vi "SEARCH DATA.vi"(11 "REFERENCES":T1) -> (3 "DATA OUT":string[][](array[string]))   [LabVIEW 2019]
uses:
  Controls/References Cluster.ctl
  Controls/Custom Calendar/Custom Calendar.xctl
  <vilib>/addons/database/Auxilliary.llb/DB Tools Cursor Type.ctl
  Controls/Column Names/Inventory Column Names.ctl
  Controls/Column Names/User Column Names.ctl
  Controls/Column Names/Inventory Archive Column Names.ctl
  Controls/Column Names/User Archive Column Names.ctl
  Controls/Column Names/Checked In Archive Column Names.ctl
  Controls/Column Names/Sales Tracking Column Names.ctl
  <vilib>/addons/database/Connection.llb/DB Tools Open Connec (String).vi
  <vilib>/addons/database/Connection.llb/Conn Execute.vi
  <vilib>/addons/database/Recordset.llb/Rec Fetch Recordset Data (R).vi
  <vilib>/addons/database/Recordset.llb/Rec Destroy - Connection.vi
  <vilib>/addons/database/_DB Variant To Data/Database Variant To Data.xnode
  <vilib>/addons/database/NI_Database_API.lvlib
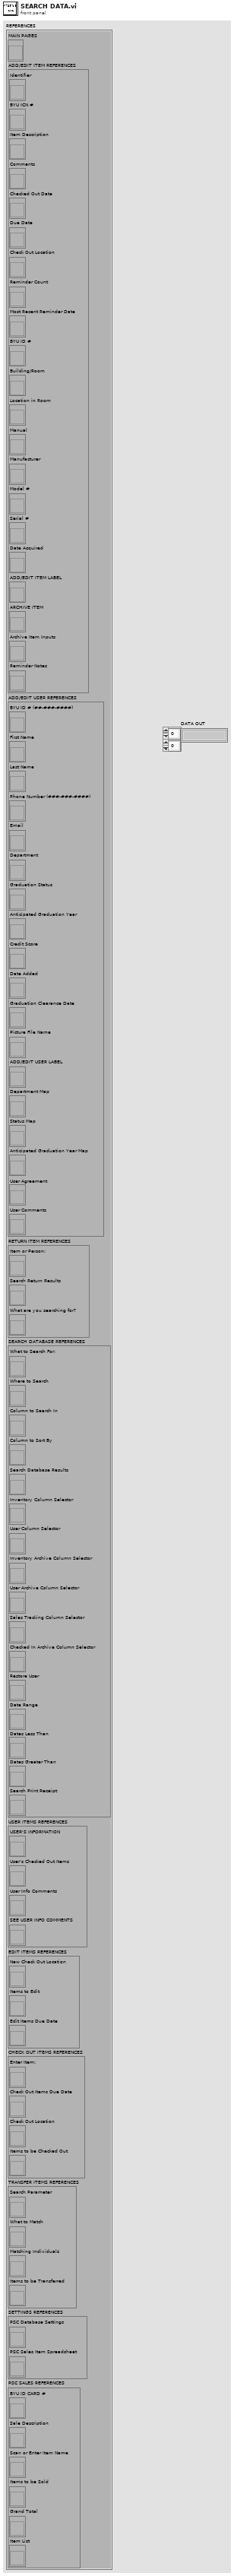
[diagram p1: front panel]
types:
  T1 = typedef "References Cluster.ctl" = cluster{"MAIN PAGES":refnum<vi>, "ADD/EDIT ITEM REFERENCES":cluster{"Identifier":refnum<vi>, "BYU ICN #":refnum<vi>, "Item Description":refnum<vi>, "Comments":refnum<vi>, "Checked Out Date":refnum<vi>, "Due Date":refnum<vi>, "Check Out Location":refnum<vi>, "Reminder Count":refnum<vi>, "Most Recent Reminder Date":refnum<vi>, "BYU ID #":refnum<vi>, "Building/Room":refnum<vi>, "Location in Room":refnum<vi>, "Manual":refnum<vi>, "Manufacturer":refnum<vi>, "Model #":refnum<vi>, "Serial #":refnum<vi>, "Date Acquired":refnum<vi>, "ADD/EDIT ITEM LABEL":refnum<vi>, "ARCHIVE ITEM":refnum<vi>, "Archive Item Inputs":refnum<vi>, "Reminder Notes":refnum<vi>}, "ADD/EDIT USER REFERENCES":cluster{"BYU ID # (##-###-####)":refnum<vi>, "First Name":refnum<vi>, "Last Name":refnum<vi>, "Phone Number (###-###-####)":refnum<vi>, "Email":refnum<vi>, "Department":refnum<vi>, "Graduation Status":refnum<vi>, "Anticipated Graduation Year":refnum<vi>, "Credit Score":refnum<vi>, "Date Added":refnum<vi>, "Graduation Clearance Date":refnum<vi>, "Picture File Name":refnum<vi>, "ADD/EDIT USER LABEL":refnum<vi>, "Department Map":refnum<vi>, "Status Map":refnum<vi>, "Anticipated Graduation Year Map":refnum<vi>, "User Agreement":refnum<vi>, "User Comments":refnum<vi>}, "RETURN ITEM REFERENCES":cluster{"Item or Person:":refnum<vi>, "Search Return Results":refnum<vi>, "What are you searching for?":refnum<vi>}, "SEARCH DATABASE REFERENCES":cluster{"What to Search For:":refnum<vi>, "Where to Search":refnum<vi>, "Column to Search In":refnum<vi>, "Column to Sort By":refnum<vi>, "Search Database Results":refnum<vi>, "Inventory Column Selector":refnum<vi>, "User Column Selector":refnum<vi>, "Inventory Archive Column Selector":refnum<vi>, "User Archive Column Selector":refnum<vi>, "Sales Tracking Column Selector":refnum<vi>, "Checked In Archive Column Selector":refnum<vi>, "Restore User":refnum<vi>, "Date Range":refnum<vi>, "Dates Less Than":refnum<vi>, "Dates Greater Than":refnum<vi>, "Search Print Receipt":refnum<vi>}, "USER ITEMS REFERENCES":cluster{"USER'S INFORMATION":refnum<vi>, "User's Checked Out Items":refnum<vi>, "User Info Comments":refnum<vi>, "SEE USER INFO COMMENTS":refnum<vi>}, "EDIT ITEMS REFERENCES":cluster{"New Check Out Location":refnum<vi>, "Items to Edit":refnum<vi>, "Edit Items Due Date":refnum<vi>}, "CHECK OUT ITEMS REFERENCES":cluster{"Enter Item:":refnum<vi>, "Check Out Items Due Date":refnum<vi>, "Check Out Location":refnum<vi>, "Items to be Checked Out":refnum<vi>}, "TRANSFER ITEMS REFERENCES":cluster{"Search Parameter":refnum<vi>, "What to Match":refnum<vi>, "Matching Individuals":refnum<vi>, "Items to be Transferred":refnum<vi>}, "SETTINGS REFERENCES":cluster{"PSC Database Settings":refnum<vi>, "PSC Sales Item Spreadsheet":refnum<vi>}, "PSC SALES REFERENCES":cluster{"BYU ID CARD #":refnum<vi>, "Sale Description":refnum<vi>, "Scan or Enter Item Name":refnum<vi>, "Items to be Sold":refnum<vi>, "Grand Total":refnum<vi>, "Item List":refnum<vi>}}
  T2 = cluster{"What to Search For:":refnum<vi>, "Where to Search":refnum<vi>, "Column to Search In":refnum<vi>, "Column to Sort By":refnum<vi>, "Search Database Results":refnum<vi>, "Inventory Column Selector":refnum<vi>, "User Column Selector":refnum<vi>, "Inventory Archive Column Selector":refnum<vi>, "User Archive Column Selector":refnum<vi>, "Sales Tracking Column Selector":refnum<vi>, "Checked In Archive Column Selector":refnum<vi>, "Restore User":refnum<vi>, "Date Range":refnum<vi>, "Dates Less Than":refnum<vi>, "Dates Greater Than":refnum<vi>, "Search Print Receipt":refnum<vi>}
  T3 = typedef "NI_Database_API.lvlib/Conn ObjectReference.ctl" = refnum<k1>
  T4 = typedef "Inventory Column Names.ctl" = string[]
  T5 = typedef "NI_Database_API.lvlib/DB Tools Cursor Type.ctl" = enum16{"forward-only", "keyset", "dynamic", "static"}
  T6 = enum8{"Enabled", "Disabled", "Disabled and Grayed Out"}
  T7 = typedef "User Column Names.ctl" = string[]
  T8 = typedef "Inventory Archive Column Names.ctl" = string[]
  T9 = typedef "User Archive Column Names.ctl" = string[]
  T10 = typedef "Checked In Archive Column Names.ctl" = string[]
  T11 = typedef "Sales Tracking Column Names.ctl" = string[]
  T12 = typedef "NI_Database_API.lvlib/Rec ObjectReference.ctl" = refnum<k1>
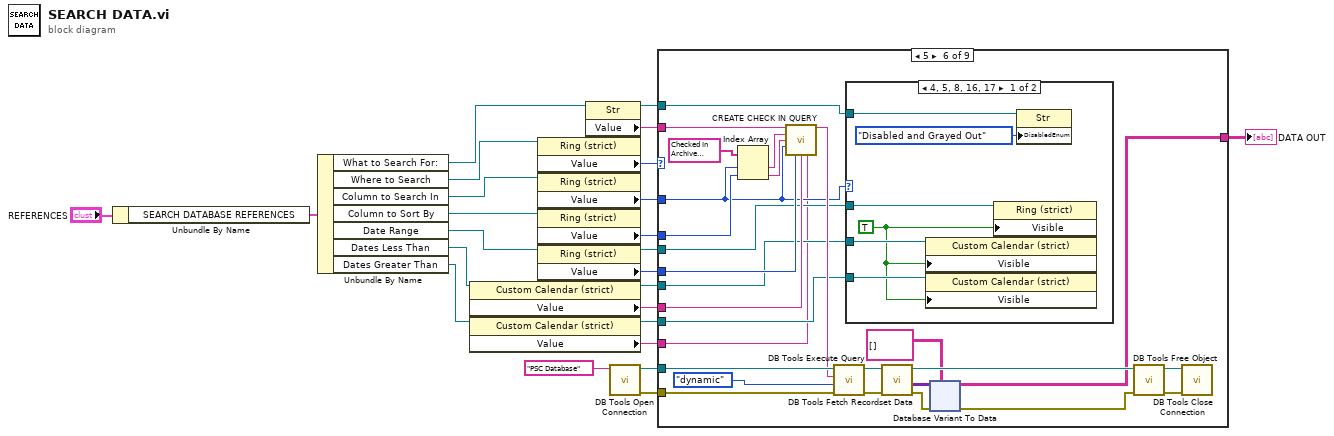
[diagram p0: block diagram]
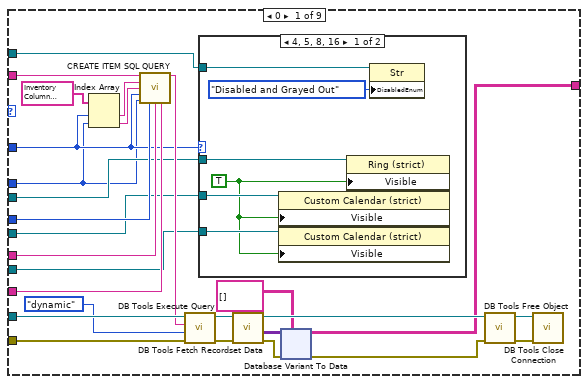
[diagram p2: hidden frame]
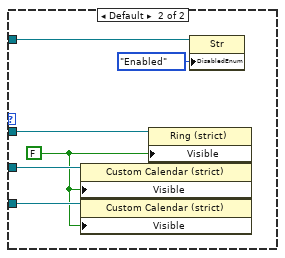
[diagram p3: hidden frame]
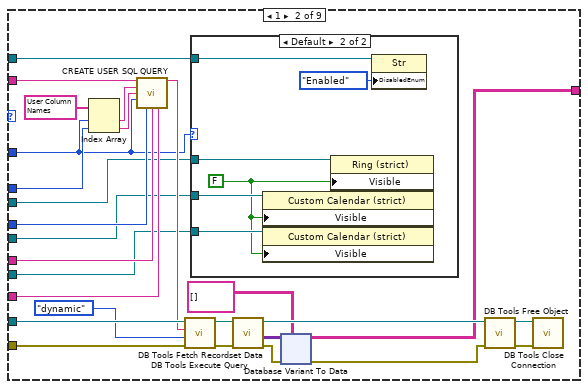
[diagram p4: hidden frame]
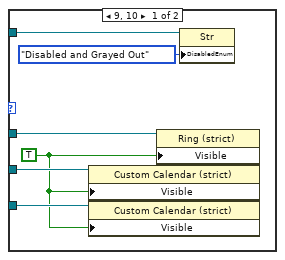
[diagram p5: hidden frame]
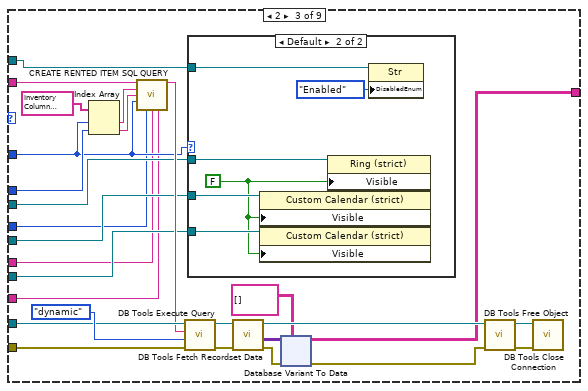
[diagram p6: hidden frame]
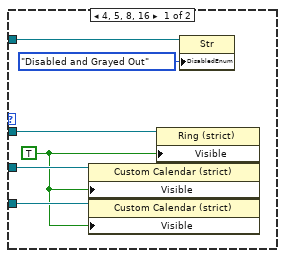
[diagram p7: hidden frame]
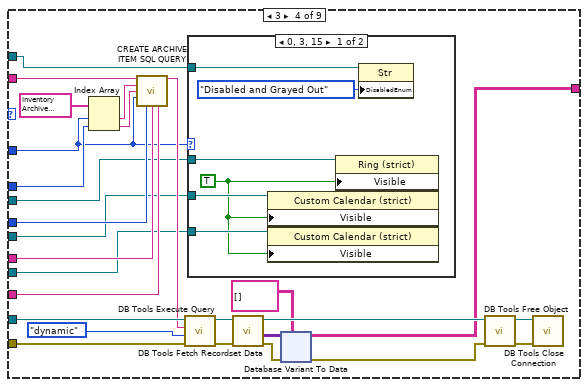
[diagram p8: hidden frame]
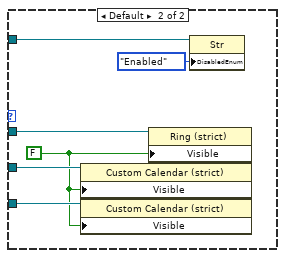
[diagram p9: hidden frame]
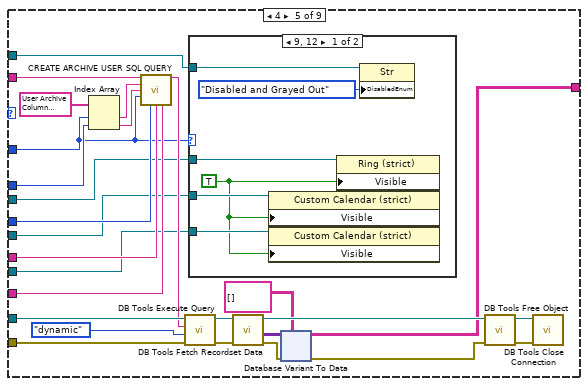
[diagram p10: hidden frame]
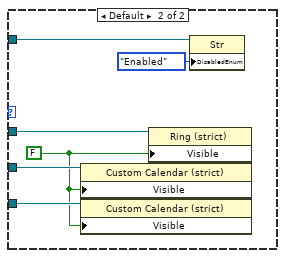
[diagram p11: hidden frame]
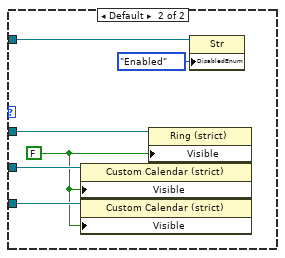
[diagram p12: hidden frame]
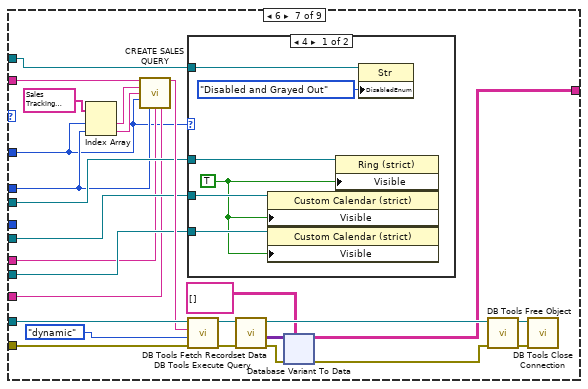
[diagram p13: hidden frame]
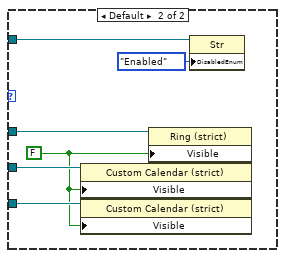
[diagram p14: hidden frame]
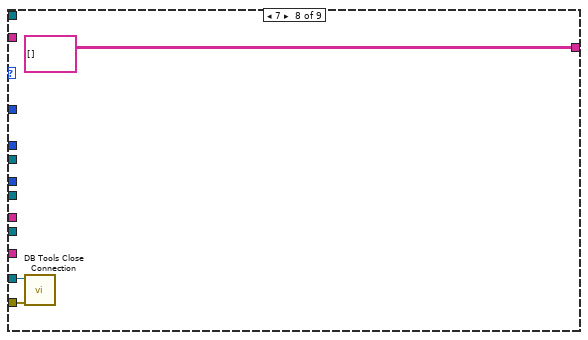
[diagram p15: hidden frame]
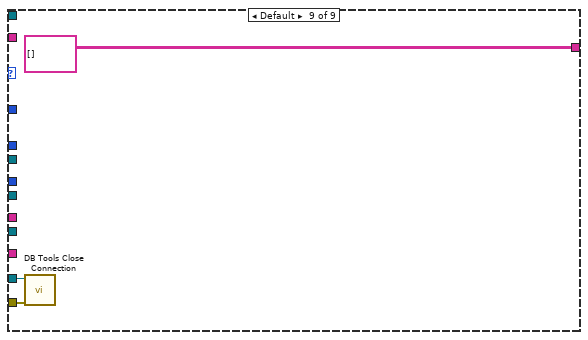
[diagram p16: hidden frame]
diagram:
  n1 = Unbundle By Name("REFERENCES") -> ("SEARCH DATABASE REFERENCES"=w13:T2)
  n2 = Unbundle By Name(w13) -> ("What to Search For:"=w18:refnum<vi>, "Where to Search"=w15:refnum<vi>, "Column to Search In"=w16:refnum<vi>, "Column to Sort By"=w17:refnum<vi>, "Date Range"=w10:refnum<vi>, "Dates Less Than"=w8:refnum<vi>, "Dates Greater Than"=w9:refnum<vi>)
  n3 = property class="Custom Calendar (strict)"(reference=w8) -> (reference out=w3:refnum<vi>, "Value"=w6:string)  [unwired: 1 in, 1 out]
  n4 = property class="Custom Calendar (strict)"(reference=w9) -> (reference out=w2:refnum<vi>, "Value"=w5:string)  [unwired: 1 in, 1 out]
  n5 = property class="Ring (strict)"(reference=w15) -> ("Value"=w24:u16)  [unwired: 1 in, 2 out]
  n6 = property class="Ring (strict)"(reference=w16) -> ("Value"=w23:u16)  [unwired: 1 in, 2 out]
  n7 = property class="Ring (strict)"(reference=w17) -> ("Value"=w22:u16)  [unwired: 1 in, 2 out]
  n8 = property class="Ring (strict)"(reference=w10) -> (reference out=w4:refnum<vi>, "Value"=w7:u16)  [unwired: 1 in, 1 out]
  n9 = property class="Str"(reference=w18) -> (reference out=w1:refnum<vi>, "Value"=w19:string)  [unwired: 1 in, 1 out]
  n10 = call-poly <vilib>:"DB Tools Open Connection.vi"("connection information"="PSC Database" ("string")) -> ("error out"=w20:errorcluster, "connection reference"=w21:T3)  [unwired: 7 in]
  n11 = case shown="5" w24 {
    tunnel: w23 -> [w31 w108 w195 w277 w361 w442 w523 _ _]
    tunnel: w22 -> [w25 w133 w217 w299 w383 w458 w526 _ _]
    tunnel: w21 -> [w51 w129 w210 w294 w376 w460 w538 w607 w610]
    tunnel: w20 -> [w50 w128 w209 w293 w375 w459 w537 w606 w609]
    tunnel: w19 -> [w43 w134 w216 w300 w382 w457 w548 _ _]
    tunnel: [w35 w118 w200 w284 w366 w450 w534 string[][] [] ("recordset data") string[][] [] ("recordset data")] -> w11
    tunnel: w7 -> [w34 w115 w194 w281 w364 w448 _ _ _]
    tunnel: w6 -> [w33 w114 w193 w280 w363 w447 w525 _ _]
    tunnel: w5 -> [w32 w113 w192 w279 w362 w441 w524 _ _]
    tunnel: w4 -> [w30 w111 w198 w276 w359 w445 w529 _ _]
    tunnel: w3 -> [w29 w110 w197 w275 w358 w444 w528 _ _]
    tunnel: w2 -> [w28 w109 w196 w274 w357 w443 w527 _ _]
    tunnel: w1 -> [w27 w112 w199 w278 w360 w446 w530 _ _]
    frame 0 {
      n12 = Index Array(array=T4 ["\"Identifier\"", "\"BYU ICN #\"", "\"Item Description\"", "\"Comments\"", "\"Checked Out Date\"", "\"Due Date\"", "\"Check Out Location\"", "\"Reminder Count\"", "\"Most Recent Reminder Date\"", "\"BYU ID #\"", "\"Building/Room\"", "\"Location in Room\"", "\"Manual\"", "\"Manufacturer\"", "\"Model #\"", "\"Serial #\"", "\"Date Acquired\"", "\"Reminder Notes\"", "\"First Name\"", "\"Last Name\""] ("INVENTORY COLUMN NAMES"), index #1=w31, index #2=w25) -> (element #1=w41:string, element #2=w40:string)
      n13 = call "CREATE ITEM SQL QUERY.vi"("What to Search"=w43, "Search Column Name"=w41, "Sorting Column Name"=w40, "Column to Search In"=w31, "Column to Sort By"=w25, "Date Range"=w34, "Dates Less Than"=w33, "Dates Greater Than"=w32) -> ("SQL QUERY"=w42:string)  [unwired: 7 in]
      n14 = call-poly <vilib>:"DB Tools Execute Query.vi"("error in (no error)"=w50, "cursor type"=DB_Tools_Cursor_Type."dynamic", "SQL query"=w42, "connection reference"=w51) -> ("error out"=w47:errorcluster, "recordset reference"=w48:T12)  [unwired: 4 in]
      n15 = case shown="4, 5, 8, 16" w31 {
        tunnel: w30 -> [w55 w61]
        tunnel: w29 -> [w56 w62]
        tunnel: w28 -> [w57 w63]
        tunnel: w27 -> [w53 w59]
        frame 4, 5, 8, 16 {
          w54 = TRUE ("Visible")
          n16 = property class="Custom Calendar (strict)"(reference=w56, "Visible"=w54) -> ()  [unwired: 1 in, 2 out]
          n17 = property class="Custom Calendar (strict)"(reference=w57, "Visible"=w54) -> ()  [unwired: 1 in, 2 out]
          n18 = property class="Ring (strict)"(reference=w55, "Visible"=w54) -> ()  [unwired: 1 in, 2 out]
          n19 = property class="Str"(reference=w53, "DisabledEnum"=T6."Disabled and Grayed Out" ("Disabled")) -> ()  [unwired: 1 in, 2 out]
        }
        frame Default {
          w58 = FALSE ("Visible")
          n20 = property class="Custom Calendar (strict)"(reference=w62, "Visible"=w58) -> ()  [unwired: 1 in, 2 out]
          n21 = property class="Custom Calendar (strict)"(reference=w63, "Visible"=w58) -> ()  [unwired: 1 in, 2 out]
          n22 = property class="Ring (strict)"(reference=w61, "Visible"=w58) -> ()  [unwired: 1 in, 2 out]
          n23 = property class="Str"(reference=w59, "DisabledEnum"=T6."Enabled" ("Disabled")) -> ()  [unwired: 1 in, 2 out]
        }
      }
      n24 = call-poly <vilib>:"DB Tools Fetch Recordset Data.vi"("error in (no error)"=w47, "recordset reference"=w48) -> ("error out"=w38:errorcluster, "recordset data"=w39:variant[][], "recordset reference out"=w46:T12)  [unwired: 3 in]
      n25 = xnode "Database Variant To Data"("database variant"=w39, "error in (no error)"=w38, "type"=string[][] []) -> ("data"=w35:string[][], "error out"=w36:errorcluster)
      n26 = call-poly <vilib>:"DB Tools Free Object.vi"("error in (no error)"=w36, "recordset reference"=w46) -> ("error out"=w44:errorcluster, "connection reference"=w45:T3)  [unwired: 8 in]
      n27 = call <vilib>:"DB Tools Close Connection.vi"("error in (no error)"=w44, "connection reference"=w45) -> ()  [unwired: 5 in, 1 out]
    }
    frame 1 {
      n28 = Index Array(array=T7 ["\"BYU ID #\"", "\"First Name\"", "\"Last Name\"", "\"Phone Number\"", "\"Email\"", "\"Department\"", "\"Graduation Status\"", "\"Anticipated Graduation Year\"", "\"Credit Score\"", "\"Date Added\"", "\"Graduation Clearance Date\"", "\"User Profile Picture Path\""] ("USER COLUMN NAMES"), index #1=w108, index #2=w133) -> (element #1=w123:string, element #2=w122:string)
      n29 = call "CREATE USER SQL QUERY.vi"("What to Search"=w134, "Search Column Name"=w123, "Sorting Column Name"=w122, "Column to Search In"=w108, "Date Range"=w115, "Dates Less Than"=w114, "Dates Greater Than"=w113) -> ("SQL QUERY"=w127:string)  [unwired: 8 in]
      n30 = call-poly <vilib>:"DB Tools Execute Query.vi"("error in (no error)"=w128, "cursor type"=DB_Tools_Cursor_Type."dynamic", "SQL query"=w127, "connection reference"=w129) -> ("error out"=w132:errorcluster, "recordset reference"=w130:T12)  [unwired: 4 in]
      n31 = case shown="Default" w108 {
        tunnel: w111 -> [w138 w144]
        tunnel: w110 -> [w139 w145]
        tunnel: w109 -> [w140 w146]
        tunnel: w112 -> [w136 w142]
        frame 9, 10 {
          w137 = TRUE ("Visible")
          n32 = property class="Custom Calendar (strict)"(reference=w139, "Visible"=w137) -> ()  [unwired: 1 in, 2 out]
          n33 = property class="Custom Calendar (strict)"(reference=w140, "Visible"=w137) -> ()  [unwired: 1 in, 2 out]
          n34 = property class="Ring (strict)"(reference=w138, "Visible"=w137) -> ()  [unwired: 1 in, 2 out]
          n35 = property class="Str"(reference=w136, "DisabledEnum"=T6."Disabled and Grayed Out" ("Disabled")) -> ()  [unwired: 1 in, 2 out]
        }
        frame Default {
          w141 = FALSE ("Visible")
          n36 = property class="Custom Calendar (strict)"(reference=w145, "Visible"=w141) -> ()  [unwired: 1 in, 2 out]
          n37 = property class="Custom Calendar (strict)"(reference=w146, "Visible"=w141) -> ()  [unwired: 1 in, 2 out]
          n38 = property class="Ring (strict)"(reference=w144, "Visible"=w141) -> ()  [unwired: 1 in, 2 out]
          n39 = property class="Str"(reference=w142, "DisabledEnum"=T6."Enabled" ("Disabled")) -> ()  [unwired: 1 in, 2 out]
        }
      }
      n40 = call-poly <vilib>:"DB Tools Fetch Recordset Data.vi"("error in (no error)"=w132, "recordset reference"=w130) -> ("error out"=w120:errorcluster, "recordset data"=w121:variant[][], "recordset reference out"=w126:T12)  [unwired: 3 in]
      n41 = xnode "Database Variant To Data"("database variant"=w121, "error in (no error)"=w120, "type"=string[][] []) -> ("data"=w118:string[][], "error out"=w117:errorcluster)
      n42 = call-poly <vilib>:"DB Tools Free Object.vi"("error in (no error)"=w117, "recordset reference"=w126) -> ("error out"=w131:errorcluster, "connection reference"=w125:T3)  [unwired: 8 in]
      n43 = call <vilib>:"DB Tools Close Connection.vi"("error in (no error)"=w131, "connection reference"=w125) -> ()  [unwired: 5 in, 1 out]
    }
    frame 2 {
      n44 = Index Array(array=T4 ["\"Identifier\"", "\"BYU ICN #\"", "\"Item Description\"", "\"Comments\"", "\"Checked Out Date\"", "\"Due Date\"", "\"Check Out Location\"", "\"Reminder Count\"", "\"Most Recent Reminder Date\"", "\"BYU ID #\"", "\"Building/Room\"", "\"Location in Room\"", "\"Manual\"", "\"Manufacturer\"", "\"Model #\"", "\"Serial #\"", "\"Date Acquired\"", "\"Reminder Notes\"", "\"First Name\"", "\"Last Name\""] ("INVENTORY COLUMN NAMES"), index #1=w195, index #2=w217) -> (element #1=w206:string, element #2=w205:string)
      n45 = call "CREATE RENTED ITEM SQL QUERY.vi"("What to Search"=w216, "Search Column Name"=w206, "Sorting Column Name"=w205, "Column to Search In"=w195, "Date Range"=w194, "Dates Less Than"=w193, "Dates Greater Than"=w192) -> ("SQL QUERY"=w208:string)  [unwired: 8 in]
      n46 = call-poly <vilib>:"DB Tools Execute Query.vi"("error in (no error)"=w209, "cursor type"=DB_Tools_Cursor_Type."dynamic", "SQL query"=w208, "connection reference"=w210) -> ("error out"=w214:errorcluster, "recordset reference"=w215:T12)  [unwired: 4 in]
      n47 = case shown="Default" w195 {
        tunnel: w198 -> [w221 w227]
        tunnel: w197 -> [w222 w228]
        tunnel: w196 -> [w223 w229]
        tunnel: w199 -> [w219 w225]
        frame 4, 5, 8, 16 {
          w220 = TRUE ("Visible")
          n48 = property class="Custom Calendar (strict)"(reference=w222, "Visible"=w220) -> ()  [unwired: 1 in, 2 out]
          n49 = property class="Custom Calendar (strict)"(reference=w223, "Visible"=w220) -> ()  [unwired: 1 in, 2 out]
          n50 = property class="Ring (strict)"(reference=w221, "Visible"=w220) -> ()  [unwired: 1 in, 2 out]
          n51 = property class="Str"(reference=w219, "DisabledEnum"=T6."Disabled and Grayed Out" ("Disabled")) -> ()  [unwired: 1 in, 2 out]
        }
        frame Default {
          w224 = FALSE ("Visible")
          n52 = property class="Custom Calendar (strict)"(reference=w228, "Visible"=w224) -> ()  [unwired: 1 in, 2 out]
          n53 = property class="Custom Calendar (strict)"(reference=w229, "Visible"=w224) -> ()  [unwired: 1 in, 2 out]
          n54 = property class="Ring (strict)"(reference=w227, "Visible"=w224) -> ()  [unwired: 1 in, 2 out]
          n55 = property class="Str"(reference=w225, "DisabledEnum"=T6."Enabled" ("Disabled")) -> ()  [unwired: 1 in, 2 out]
        }
      }
      n56 = call-poly <vilib>:"DB Tools Fetch Recordset Data.vi"("error in (no error)"=w214, "recordset reference"=w215) -> ("error out"=w203:errorcluster, "recordset data"=w204:variant[][], "recordset reference out"=w213:T12)  [unwired: 3 in]
      n57 = xnode "Database Variant To Data"("database variant"=w204, "error in (no error)"=w203, "type"=string[][] []) -> ("data"=w200:string[][], "error out"=w202:errorcluster)
      n58 = call-poly <vilib>:"DB Tools Free Object.vi"("error in (no error)"=w202, "recordset reference"=w213) -> ("error out"=w212:errorcluster, "connection reference"=w207:T3)  [unwired: 8 in]
      n59 = call <vilib>:"DB Tools Close Connection.vi"("error in (no error)"=w212, "connection reference"=w207) -> ()  [unwired: 5 in, 1 out]
    }
    frame 3 {
      n60 = Index Array(array=T8 ["\"Date Disposed\"", "\"Disposal Method\"", "\"Auction #\"", "\"Date Inventory Office Emailed\"", "\"Disposal Notes\"", "\"Identifier\"", "\"BYU ICN #\"", "\"Item Description\"", "\"Comments\"", "\"Building/Room\"", "\"Location in Room\"", "\"Manual\"", "\"Manufacturer\"", "\"Model #\"", "\"Serial #\"", "\"Date Acquired\""] ("INVENTORY ARCHIVE COLUMN NAMES"), index #1=w277, index #2=w299) -> (element #1=w289:string, element #2=w288:string)
      n61 = call "CREATE ARCHIVE ITEM SQL QUERY.vi"("What to Search"=w300, "Search Column Name"=w289, "Sorting Column Name"=w288, "Column to Search In"=w277, "Date Range"=w281, "Dates Less Than"=w280, "Dates Greater Than"=w279) -> ("SQL QUERY"=w292:string)  [unwired: 8 in]
      n62 = call-poly <vilib>:"DB Tools Execute Query.vi"("error in (no error)"=w293, "cursor type"=DB_Tools_Cursor_Type."dynamic", "SQL query"=w292, "connection reference"=w294) -> ("error out"=w297:errorcluster, "recordset reference"=w298:T12)  [unwired: 4 in]
      n63 = case shown="0, 3, 15" w277 {
        tunnel: w276 -> [w304 w310]
        tunnel: w275 -> [w305 w311]
        tunnel: w274 -> [w306 w312]
        tunnel: w278 -> [w302 w308]
        frame 0, 3, 15 {
          w303 = TRUE ("Visible")
          n64 = property class="Custom Calendar (strict)"(reference=w305, "Visible"=w303) -> ()  [unwired: 1 in, 2 out]
          n65 = property class="Custom Calendar (strict)"(reference=w306, "Visible"=w303) -> ()  [unwired: 1 in, 2 out]
          n66 = property class="Ring (strict)"(reference=w304, "Visible"=w303) -> ()  [unwired: 1 in, 2 out]
          n67 = property class="Str"(reference=w302, "DisabledEnum"=T6."Disabled and Grayed Out" ("Disabled")) -> ()  [unwired: 1 in, 2 out]
        }
        frame Default {
          w307 = FALSE ("Visible")
          n68 = property class="Custom Calendar (strict)"(reference=w311, "Visible"=w307) -> ()  [unwired: 1 in, 2 out]
          n69 = property class="Custom Calendar (strict)"(reference=w312, "Visible"=w307) -> ()  [unwired: 1 in, 2 out]
          n70 = property class="Ring (strict)"(reference=w310, "Visible"=w307) -> ()  [unwired: 1 in, 2 out]
          n71 = property class="Str"(reference=w308, "DisabledEnum"=T6."Enabled" ("Disabled")) -> ()  [unwired: 1 in, 2 out]
        }
      }
      n72 = call-poly <vilib>:"DB Tools Fetch Recordset Data.vi"("error in (no error)"=w297, "recordset reference"=w298) -> ("error out"=w285:errorcluster, "recordset data"=w286:variant[][], "recordset reference out"=w291:T12)  [unwired: 3 in]
      n73 = xnode "Database Variant To Data"("database variant"=w286, "error in (no error)"=w285, "type"=string[][] []) -> ("data"=w284:string[][], "error out"=w283:errorcluster)
      n74 = call-poly <vilib>:"DB Tools Free Object.vi"("error in (no error)"=w283, "recordset reference"=w291) -> ("error out"=w296:errorcluster, "connection reference"=w290:T3)  [unwired: 8 in]
      n75 = call <vilib>:"DB Tools Close Connection.vi"("error in (no error)"=w296, "connection reference"=w290) -> ()  [unwired: 5 in, 1 out]
    }
    frame 4 {
      n76 = Index Array(array=T9 ["\"BYU ID #\"", "\"First Name\"", "\"Last Name\"", "\"Phone Number\"", "\"Email\"", "\"Department\"", "\"Graduation Status\"", "\"Anticipated Graduation Year\"", "\"Credit Score\"", "\"Date Added\"", "\"Graduation Clearance Date\"", "\"Picture File Name\"", "\"Date Archived\""] ("USER ARCHIVE COLUMN NAMES"), index #1=w361, index #2=w383) -> (element #1=w372:string, element #2=w371:string)
      n77 = call "CREATE ARCHIVE USER SQL QUERY.vi"("What to Search"=w382, "Search Column Name"=w372, "Sorting Column Name"=w371, "Column to Search In"=w361, "Date Range"=w364, "Dates Less Than"=w363, "Dates Greater Than"=w362) -> ("SQL QUERY"=w374:string)  [unwired: 8 in]
      n78 = call-poly <vilib>:"DB Tools Execute Query.vi"("error in (no error)"=w375, "cursor type"=DB_Tools_Cursor_Type."dynamic", "SQL query"=w374, "connection reference"=w376) -> ("error out"=w380:errorcluster, "recordset reference"=w381:T12)  [unwired: 4 in]
      n79 = case shown="9, 12" w361 {
        tunnel: w359 -> [w387 w393]
        tunnel: w358 -> [w388 w394]
        tunnel: w357 -> [w389 w395]
        tunnel: w360 -> [w385 w391]
        frame 9, 12 {
          w386 = TRUE ("Visible")
          n80 = property class="Custom Calendar (strict)"(reference=w388, "Visible"=w386) -> ()  [unwired: 1 in, 2 out]
          n81 = property class="Custom Calendar (strict)"(reference=w389, "Visible"=w386) -> ()  [unwired: 1 in, 2 out]
          n82 = property class="Ring (strict)"(reference=w387, "Visible"=w386) -> ()  [unwired: 1 in, 2 out]
          n83 = property class="Str"(reference=w385, "DisabledEnum"=T6."Disabled and Grayed Out" ("Disabled")) -> ()  [unwired: 1 in, 2 out]
        }
        frame Default {
          w390 = FALSE ("Visible")
          n84 = property class="Custom Calendar (strict)"(reference=w394, "Visible"=w390) -> ()  [unwired: 1 in, 2 out]
          n85 = property class="Custom Calendar (strict)"(reference=w395, "Visible"=w390) -> ()  [unwired: 1 in, 2 out]
          n86 = property class="Ring (strict)"(reference=w393, "Visible"=w390) -> ()  [unwired: 1 in, 2 out]
          n87 = property class="Str"(reference=w391, "DisabledEnum"=T6."Enabled" ("Disabled")) -> ()  [unwired: 1 in, 2 out]
        }
      }
      n88 = call-poly <vilib>:"DB Tools Fetch Recordset Data.vi"("error in (no error)"=w380, "recordset reference"=w381) -> ("error out"=w369:errorcluster, "recordset data"=w370:variant[][], "recordset reference out"=w378:T12)  [unwired: 3 in]
      n89 = xnode "Database Variant To Data"("database variant"=w370, "error in (no error)"=w369, "type"=string[][] []) -> ("data"=w366:string[][], "error out"=w368:errorcluster)
      n90 = call-poly <vilib>:"DB Tools Free Object.vi"("error in (no error)"=w368, "recordset reference"=w378) -> ("error out"=w379:errorcluster, "connection reference"=w377:T3)  [unwired: 8 in]
      n91 = call <vilib>:"DB Tools Close Connection.vi"("error in (no error)"=w379, "connection reference"=w377) -> ()  [unwired: 5 in, 1 out]
    }
    frame 5 {
      n92 = Index Array(array=T10 ["\"Identifier\"", "\"BYU ICN #\"", "\"Item Description\"", "\"Comments\"", "\"Checked Out Date\"", "\"Due Date\"", "\"Check Out Location\"", "\"Reminder Count\"", "\"Most Recent Reminder Date\"", "\"BYU ID #\"", "\"Building/Room\"", "\"Location in Room\"", "\"Manual\"", "\"Manufacturer\"", "\"Model #\"", "\"Serial #\"", "\"Date Acquired\"", "\"Date Returned\"", "\"Reminder Notes\"", "\"First Name\"", "\"Last Name\""] ("CHECKED IN ARCHIVE COLUMN NAMES"), index #1=w442, index #2=w458) -> (element #1=w456:string, element #2=w455:string)
      n93 = call "CREATE CHECK IN QUERY.vi"("What to Search"=w457, "Search Column Name"=w456, "Sorting Column Name"=w455, "Column to Search In"=w442, "Date Range"=w448, "Dates Less Than"=w447, "Dates Greater Than"=w441) -> ("SQL QUERY"=w454:string)  [unwired: 8 in]
      n94 = call-poly <vilib>:"DB Tools Execute Query.vi"("error in (no error)"=w459, "cursor type"=DB_Tools_Cursor_Type."dynamic", "SQL query"=w454, "connection reference"=w460) -> ("error out"=w465:errorcluster, "recordset reference"=w466:T12)  [unwired: 4 in]
      n95 = case shown="4, 5, 8, 16, 17" w442 {
        tunnel: w445 -> [w470 w476]
        tunnel: w444 -> [w471 w477]
        tunnel: w443 -> [w472 w478]
        tunnel: w446 -> [w468 w474]
        frame 4, 5, 8, 16, 17 {
          w469 = TRUE ("Visible")
          n96 = property class="Custom Calendar (strict)"(reference=w471, "Visible"=w469) -> ()  [unwired: 1 in, 2 out]
          n97 = property class="Custom Calendar (strict)"(reference=w472, "Visible"=w469) -> ()  [unwired: 1 in, 2 out]
          n98 = property class="Ring (strict)"(reference=w470, "Visible"=w469) -> ()  [unwired: 1 in, 2 out]
          n99 = property class="Str"(reference=w468, "DisabledEnum"=T6."Disabled and Grayed Out" ("Disabled")) -> ()  [unwired: 1 in, 2 out]
        }
        frame Default {
          w473 = FALSE ("Visible")
          n100 = property class="Custom Calendar (strict)"(reference=w477, "Visible"=w473) -> ()  [unwired: 1 in, 2 out]
          n101 = property class="Custom Calendar (strict)"(reference=w478, "Visible"=w473) -> ()  [unwired: 1 in, 2 out]
          n102 = property class="Ring (strict)"(reference=w476, "Visible"=w473) -> ()  [unwired: 1 in, 2 out]
          n103 = property class="Str"(reference=w474, "DisabledEnum"=T6."Enabled" ("Disabled")) -> ()  [unwired: 1 in, 2 out]
        }
      }
      n104 = call-poly <vilib>:"DB Tools Fetch Recordset Data.vi"("error in (no error)"=w465, "recordset reference"=w466) -> ("error out"=w452:errorcluster, "recordset data"=w453:variant[][], "recordset reference out"=w463:T12)  [unwired: 3 in]
      n105 = xnode "Database Variant To Data"("database variant"=w453, "error in (no error)"=w452, "type"=string[][] []) -> ("data"=w450:string[][], "error out"=w451:errorcluster)
      n106 = call-poly <vilib>:"DB Tools Free Object.vi"("error in (no error)"=w451, "recordset reference"=w463) -> ("error out"=w464:errorcluster, "connection reference"=w462:T3)  [unwired: 8 in]
      n107 = call <vilib>:"DB Tools Close Connection.vi"("error in (no error)"=w464, "connection reference"=w462) -> ()  [unwired: 5 in, 1 out]
    }
    frame 6 {
      n108 = Index Array(array=T11 ["\"SALE ID #\"", "\"BYU ID CARD #\"", "\"Sale Description\"", "\"Grand Total\"", "\"Sale Date\"", "\"Item Description\"", "\"Item Quantity\"", "\"Item Unit Price\"", "\"Item Total Price\"", "\"Sale Semester\""] ("Sales Tracking Column Names"), index #1=w523, index #2=w526) -> (element #1=w547:string, element #2=w546:string)
      n109 = call "CREATE SALES QUERY.vi"("What to Search"=w548, "Search Column Name"=w547, "Sorting Column Name"=w546, "Column to Search In"=w523, "Date Range"=w526, "Dates Less Than"=w525, "Dates Greater Than"=w524) -> ("SQL QUERY"=w533:string)  [unwired: 8 in]
      n110 = case shown="4" w523 {
        tunnel: w529 -> [w552 w558]
        tunnel: w528 -> [w553 w559]
        tunnel: w527 -> [w554 w560]
        tunnel: w530 -> [w550 w556]
        frame 4 {
          w551 = TRUE ("Visible")
          n111 = property class="Custom Calendar (strict)"(reference=w553, "Visible"=w551) -> ()  [unwired: 1 in, 2 out]
          n112 = property class="Custom Calendar (strict)"(reference=w554, "Visible"=w551) -> ()  [unwired: 1 in, 2 out]
          n113 = property class="Ring (strict)"(reference=w552, "Visible"=w551) -> ()  [unwired: 1 in, 2 out]
          n114 = property class="Str"(reference=w550, "DisabledEnum"=T6."Disabled and Grayed Out" ("Disabled")) -> ()  [unwired: 1 in, 2 out]
        }
        frame Default {
          w555 = FALSE ("Visible")
          n115 = property class="Custom Calendar (strict)"(reference=w559, "Visible"=w555) -> ()  [unwired: 1 in, 2 out]
          n116 = property class="Custom Calendar (strict)"(reference=w560, "Visible"=w555) -> ()  [unwired: 1 in, 2 out]
          n117 = property class="Ring (strict)"(reference=w558, "Visible"=w555) -> ()  [unwired: 1 in, 2 out]
          n118 = property class="Str"(reference=w556, "DisabledEnum"=T6."Enabled" ("Disabled")) -> ()  [unwired: 1 in, 2 out]
        }
      }
      n119 = call-poly <vilib>:"DB Tools Execute Query.vi"("error in (no error)"=w537, "cursor type"=DB_Tools_Cursor_Type."dynamic", "SQL query"=w533, "connection reference"=w538) -> ("error out"=w544:errorcluster, "recordset reference"=w545:T12)  [unwired: 4 in]
      n120 = call-poly <vilib>:"DB Tools Fetch Recordset Data.vi"("error in (no error)"=w544, "recordset reference"=w545) -> ("error out"=w541:errorcluster, "recordset data"=w542:variant[][], "recordset reference out"=w543:T12)  [unwired: 3 in]
      n121 = xnode "Database Variant To Data"("database variant"=w542, "error in (no error)"=w541, "type"=string[][] []) -> ("data"=w534:string[][], "error out"=w540:errorcluster)
      n122 = call-poly <vilib>:"DB Tools Free Object.vi"("error in (no error)"=w540, "recordset reference"=w543) -> ("error out"=w535:errorcluster, "connection reference"=w536:T3)  [unwired: 8 in]
      n123 = call <vilib>:"DB Tools Close Connection.vi"("error in (no error)"=w535, "connection reference"=w536) -> ()  [unwired: 5 in, 1 out]
    }
    frame 7 {
      n124 = call <vilib>:"DB Tools Close Connection.vi"("error in (no error)"=w606, "connection reference"=w607) -> ()  [unwired: 5 in, 1 out]
    }
    frame Default {
      n125 = call <vilib>:"DB Tools Close Connection.vi"("error in (no error)"=w609, "connection reference"=w610) -> ()  [unwired: 5 in, 1 out]
    }
  }
  "DATA OUT" <- w11
